vi "Set IPS Action.vi"(8 "error in (no error)":errorcluster, 10 "PSU Act Stat":T1="HOLD" caption="PSU Action Status", 11 "Instrument.Oxford1820 in":refnum<class "Instrument.Oxford1820.lvclass">) -> (0 "error out":errorcluster, 2 "Response":string, 3 "Instrument.Oxford1820 out":refnum<class "Instrument.Oxford1820.lvclass">)   [LabVIEW 2016, in "Instrument.Oxford1820.lvclass"]
uses:
  Instrument.Oxford1820.lvclass
  <instrlib>/Mercury iXX/Public/Libraries/Magnet/Controls/PSU Actions.ctl
  Instrument.Oxford1820.lvclass/Instrument.Oxford1820.ctl
  <instrlib>/Mercury iXX/Public/Libraries/Magnet/Open/Open Magnet Device.vi
  <instrlib>/Mercury iXX/Public/Libraries/Magnet/Configuration/Set/PSU Action Status (Set).vi
  <instrlib>/Mercury iXX/Public/Libraries/Magnet/Configuration/Read/PSU Action Status (Read).vi
  <instrlib>/Mercury iXX/Mercury iXX.lvlib
  <instrlib>/Mercury iXX/Public/Libraries/Magnet.lvlib
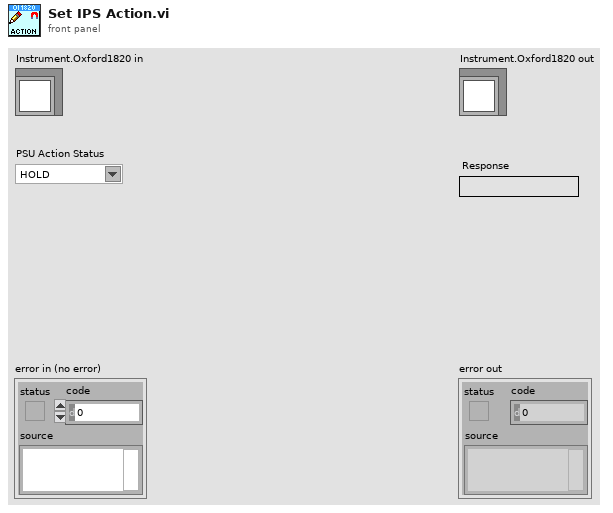
[diagram p1: front panel]
types:
  T1 = typedef "Mercury iXX.lvlib/Magnet.lvlib/PSU Actions.ctl" = string
  T2 = typedef "Mercury iXX.lvlib/Mercury Reference.ctl" = cluster{"Comms":refnum<visa-resource-name>, "Device ID":string[], "Comms Layer":T3, "Command":string, "Query reference":T4}
  T3 = typedef "Mercury iXX.lvlib/Comms Transport Layer.ctl" = enum16{"Ethernet TCP/IP", "USB", "ISOBus - RS-232", "GPIB"}
  T4 = typedef "Mercury iXX.lvlib/Query Dynamic Reference.ctl" = refnum<vi>
  T5 = typedef "Mercury iXX.lvlib/Response String.ctl" = string
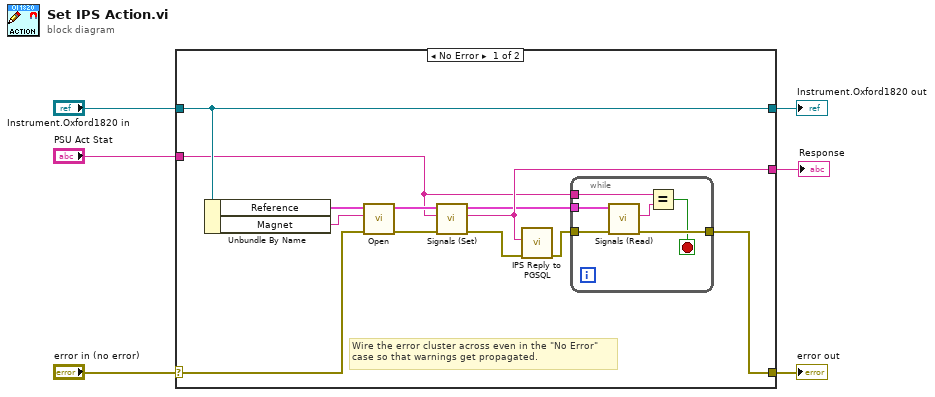
[diagram p0: block diagram]
diagram:
  n1 = case shown="No Error" "error in (no error)" {
    selector: "error in (no error)" -> [w15 w26]
    tunnel: [w9 w26] -> w5
    tunnel: [w18 w25] -> w3
    tunnel: "Instrument.Oxford1820 in" -> [w18 w25]
    tunnel: [w11 _] -> w2
    tunnel: "PSU Act Stat" -> [w8 _]
    frame No Error {
      # "Wire the error cluster across even in the \"No Error\"\ncase so that warnings get propagated."
      n2 = Unbundle By Name(w18) -> ("Reference"=w16:T2, "Magnet"=w17:string)
      n3 = call-poly <instrlib>:"Open.vi"("error in (no error)"=w15, "Device Identifier"=w17, "Mercury Reference In"=w16) -> ("error out"=w13:errorcluster, "Mercury Reference Out"=w14:T2)  [unwired: 7 out]
      n4 = call-poly <instrlib>:"Signals (Set).vi"("error in"=w13, "PSU Act Stat"=w8, "Mercury Reference In"=w14) -> ("error out"=w12:errorcluster, "Response"=w11:T5, "Mercury Reference Out"=w10:T2)  [unwired: 1 in, 5 out]
      n5 = call "IPS Reply to PGSQL.vi"("error in (no error)"=w12, "Response"=w11) -> ("error out"=w7:errorcluster)  [unwired: 9 in]
      n6 = while {
        tunnel: w7 -> [w23]
        tunnel: w10 -> [w24]
        tunnel: [w22] -> w9
        tunnel: w8 -> [w21]
        stop <- w19 stop-if-true
        n7 = call-poly <instrlib>:"Signals (Read).vi"("error in"=w23, "Mercury Reference In"=w24) -> ("error out"=w22:errorcluster, "PSU Act Stat"=w20:T1)  [unwired: 1 in, 7 out]
        n8 = Equal?(x=w21, y=w20) -> (x = y?=w19:bool)
      }
    }
    frame Error {
    }
  }
  "error out" <- w5
  "Instrument.Oxford1820 out" <- w3
  "Response" <- w2
